vi "Read Array of Device Configuration.vi"(8 "error in (no error)":errorcluster, 11 "Measurement Data in":refnum<class "Measurement Data.lvclass">) -> (0 "error out":errorcluster, 2 "Array of Device Configuration":refnum<class "HW Configuration.lvclass">[](array[class]), 3 "Measurement Data out":refnum<class "Measurement Data.lvclass">)   [LabVIEW 2016, in "Measurement Setup Controller.lvlib" / "Measurement Data.lvclass"]
uses:
  Measurement Data.lvclass
  MAL-Framework/user.lib/Common Components/Hardware/HW Config/HW Configuration.lvclass
  Measurement Data.lvclass/Measurement Data.ctl
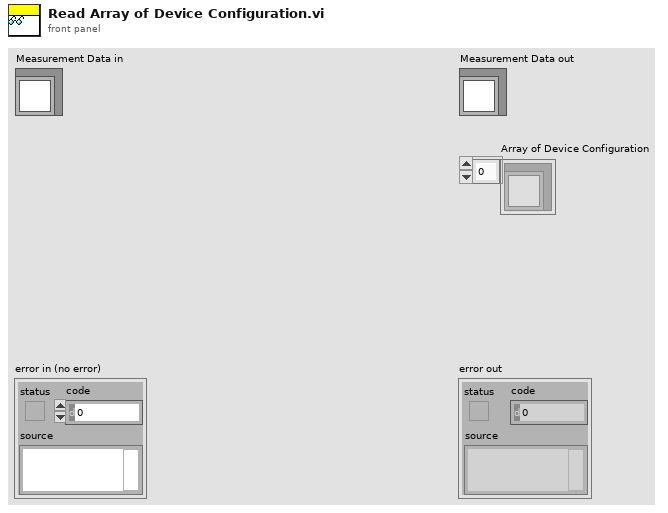
[diagram p1: front panel]
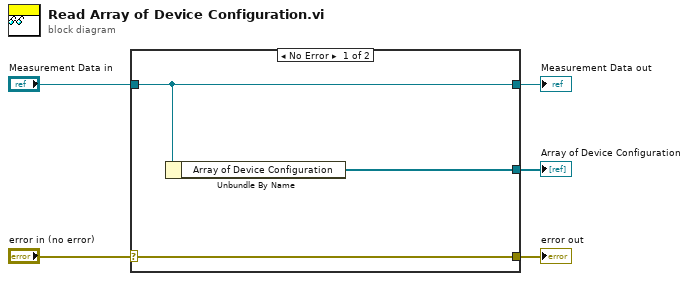
[diagram p0: block diagram]
diagram:
  n1 = case shown="No Error" "error in (no error)" {
    selector: "error in (no error)" -> [w8 w9]
    tunnel: [w8 w9] -> w4
    tunnel: [w7 w10] -> w2
    tunnel: "Measurement Data in" -> [w7 w10]
    tunnel: [w6 _] -> w1
    frame No Error {
      n2 = Unbundle By Name(w7) -> ("Array of Device Configuration"=w6:refnum<class "HW Configuration.lvclass">[])
    }
    frame Error {
    }
  }
  "error out" <- w4
  "Measurement Data out" <- w2
  "Array of Device Configuration" <- w1
